vi "Get Display Data.vi"(8 "error in (no error)":errorcluster, 11 "Standard Display Configuration in":refnum<class "Standard Display Configuration.lvclass">) -> (0 "error out":errorcluster, 2 "Display Data":string[][](array[string]))   [LabVIEW 2016, in "Assert API Components.lvlib" / "Assert Display.lvlib" / "Main Display.lvlib" / "Standard Display Configuration.lvclass"]
uses:
  Standard Display Configuration.lvclass
  D:/Work/Projects/Actor_Assert_API/Main Display/Display Configurations/Base Display Configuration.lvclass
  Base Display Configuration.lvclass/Base Display Configuration.ctl
  Base Display Configuration.lvclass
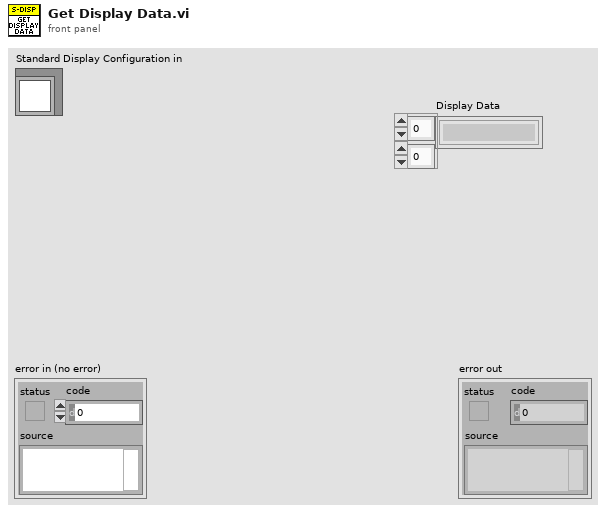
[diagram p1: front panel]
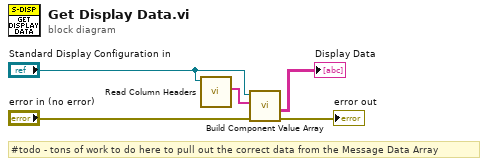
[diagram p0: block diagram]
diagram:
  # "#todo - tons of work to do here to pull out the correct data from the Message Data Array"
  n1 = call "Read Column Headers.vi"("Base Display Configuration in"="Standard Display Configuration in") -> ("Column Headers"=w1:string[])  [unwired: 10 in]
  n2 = call "Build Component Value Array.vi"("error in (no error)"="error in (no error)", "Component Name Array"=w1, "Standard Display Configuration in"="Standard Display Configuration in") -> ("error out"=→"error out":errorcluster, "Component Value Array"=→"Display Data":string[][])  [unwired: 7 in]
